vi "GUI Write Sequence Item Status.vi"(4 "multiplex enabled (False)":bool, 6 "multiplex tag":string, 7 "status label":string="stat2", 8 "error in":errorcluster, 9 "sub-rec id":i32, 10 "sub-rec count":i32=1, 11 "sequence item":T1) -> (0 "error out":errorcluster, 3 "sequence item (copy)":T1)   [LabVIEW 2020]
doc: "Updates measurement status for each sequence item. Can generate error, but will exdcute even with input error."
uses:
  Meas Sequence Item.ctl
  Meas Sampling Configuration.ctl
  adc/ADC Trig Config.ctl
  adc/ADC Trig Mode Source.ctl
  adc/ADC Trig Slope.ctl
  adc/ADC Trig Coupling.ctl
  processing/QWTB/Meas Proc QWTB Algorithm Parameter Data.ctl
  drivers/DMM/3458A Sampling Rate.ctl
  drivers/AWG/AWG Clock Setup Mode.ctl
  varilib/SGUI Assign Multiple Strings With Tags By Label.vi
  varilib/varilib.lvlib
  drivers/AWG/AWG.lvlib
  drivers/DMM/3458A Virtual Digitizer.lvlib
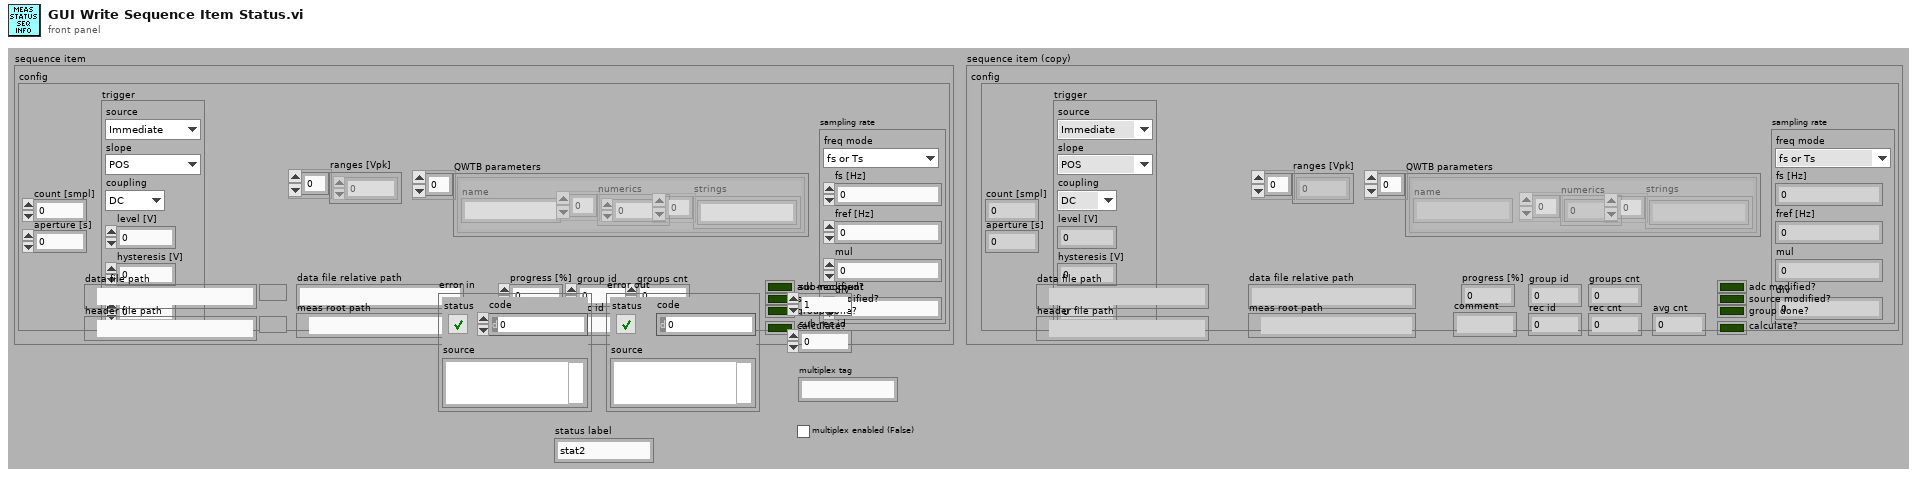
[diagram p1: front panel]
types:
  T1 = typedef "Meas Sequence Item.ctl" = cluster{"config":T2, "data file path":path, "header file path":path, "group id":i32, "rec id":i32, "group done?":bool, "adc modified?":bool, "source modified?":bool, "progress [%]":dbl, "groups cnt":i32, "rec cnt":i32, "data file relative path":string, "meas root path":path, "calculate?":bool, "comment":string, "avg cnt":i32}
  T2 = typedef "Meas Sampling Configuration.ctl" = cluster{"count [smpl]":i64, "aperture [s]":dbl, "trigger":T3, "ranges [Vpk]":dbl[], "QWTB parameters":T7[], "sampling rate":T8}
  T3 = typedef "ADC Trig Config.ctl" = cluster{"source":T4, "slope":T5, "coupling":T6, "level [V]":dbl, "hysteresis [V]":dbl, "pre-trigger [%]":dbl}
  T4 = typedef "ADC Trig Mode Source.ctl" = enum16{"Immediate", "External", "Level"}
  T5 = typedef "ADC Trig Slope.ctl" = enum16{"POS", "NEG"}
  T6 = typedef "ADC Trig Coupling.ctl" = enum16{"DC", "AC"}
  T7 = typedef "Meas Proc QWTB Algorithm Parameter Data.ctl" = cluster{"name":string, "numerics":dbl[], "strings":string[]}
  T8 = typedef "3458A Virtual Digitizer.lvlib/3458A Sampling Rate.ctl" = cluster{"freq mode":T9, "fs [Hz]":dbl, "fref [Hz]":dbl, "mul":dbl, "div":dbl}
  T9 = typedef "AWG.lvlib/AWG Clock Setup Mode.ctl" = enum16{"fs or Ts", "fs or Ts with fref", "fref/N", "fref*M/N", "fref*Ratio"}
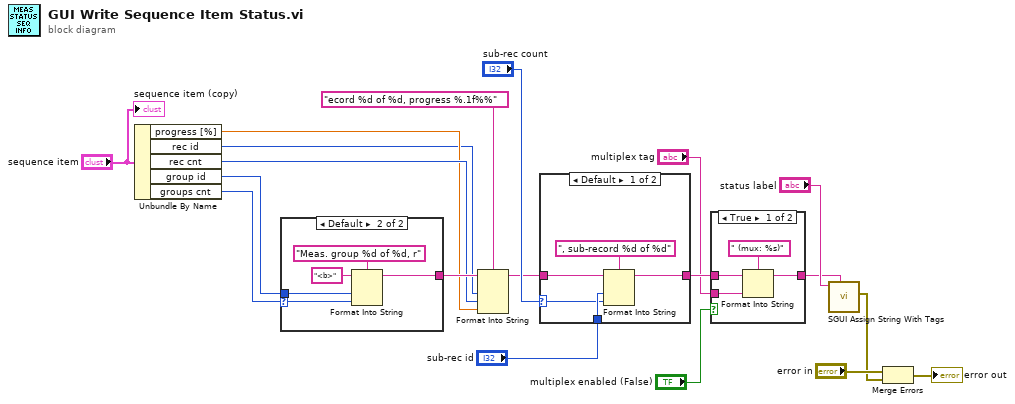
[diagram p0: block diagram]
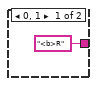
[diagram p4: hidden frame]
diagram:
  n1 = Unbundle By Name("sequence item") -> ("progress [%]"=w14:dbl, "rec id"=w8:i32, "rec cnt"=w15:i32, "group id"=w18:i32, "groups cnt"=w17:i32)
  n2 = case shown="Default" w17 {
    selector: w17 -> [_ w24]
    tunnel: w18 -> [_ w22]
    tunnel: ["<b>R" w23] -> w16
    frame 0, 1 {
    }
    frame Default {
      n3 = Format Into String(format string="Meas. group %d of %d, r", initial string="<b>", w22, w24) -> (resulting string=w23:string)  [unwired: 1 in, 1 out]
    }
  }
  n4 = Format Into String(format string="ecord %d of %d, progress %.1f%%", initial string=w16, w8, w15, w14) -> (resulting string=w6:string)  [unwired: 1 in, 1 out]
  n5 = case shown="Default" "sub-rec count" {
    selector: "sub-rec count" -> [w27 _]
    tunnel: w6 -> [w30 w31]
    tunnel: "sub-rec id" -> [w28 _]
    tunnel: [w26 w31] -> w4
    frame Default {
      n6 = Format Into String(format string=", sub-record %d of %d", initial string=w30, w28, w27) -> (resulting string=w26:string)  [unwired: 1 in, 1 out]
    }
    frame 0, 1 {
    }
  }
  n7 = case shown="True" "multiplex enabled (False)" {
    tunnel: w4 -> [w35 w36]
    tunnel: [w33 w36] -> w1
    tunnel: "multiplex tag" -> [w32 _]
    frame True {
      n8 = Format Into String(format string=" (mux: %s)", initial string=w35, w32) -> (resulting string=w33:string)  [unwired: 1 in, 1 out]
    }
    frame False {
    }
  }
  n9 = call-poly "SGUI Assign String With Tags.vi"("label(s) (empty)"="status label", "string (empty)"=w1) -> ("error out"=w10:errorcluster)  [unwired: 8 in, 1 out]
  n10 = Merge Errors("error in", w10) -> (→"error out":errorcluster)
  "sequence item (copy)" <- "sequence item"
